vi "Wait.Gui.Open.vi"(6 "Delay at open [ms]":u32, 8 "error in (no error)":errorcluster, 9 "ProgBarSize (0)":i32, 10 "Status (\"\")":string, 11 "Msg":string) -> (0 "error out":errorcluster)   [LabVIEW 2016]
uses:
  Wait.Gui.Action.ctl
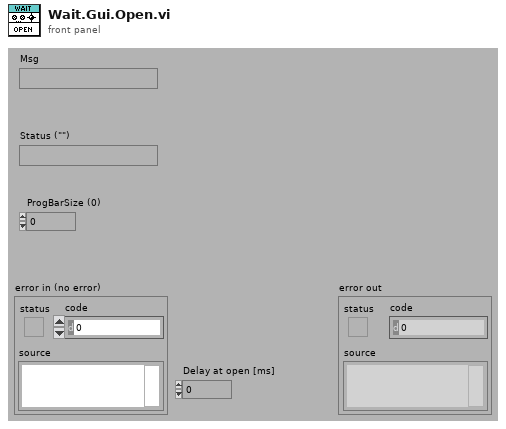
[diagram p1: front panel]
types:
  T1 = typedef "Wait.Gui.Action.ctl" = enum32{"idle", "constructor", "destructor", "--- WaitGui ---", "open FP", "close FP", "update msg", "update progbar"}
  T2 = cluster{"Msg":string, "Status (\"\")":string, "ProgBarSize (0)":i32, "Delay at open [ms]":u32}
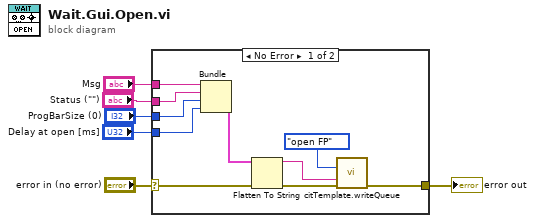
[diagram p0: block diagram]
diagram:
  n1 = case shown="No Error" "error in (no error)" {
    selector: "error in (no error)" -> [w9 w17]
    tunnel: [w16 w17] -> w6
    tunnel: "Msg" -> [w12 _]
    tunnel: "Status (\"\")" -> [w11 _]
    tunnel: "ProgBarSize (0)" -> [w8 _]
    tunnel: "Delay at open [ms]" -> [w7 _]
    frame No Error {
      n2 = Bundle("Msg"=w12, "Status (\"\")"=w11, "ProgBarSize (0)"=w8, "Delay at open [ms]"=w7) -> (w10:T2)  [unwired: 1 in]
      n3 = Flatten To String(anything=w10, error in (no error)=w9) -> (data string=w14:string, error out=w13:errorcluster)  [unwired: 2 in, 1 out]
      n4 = call "citTemplate.writeQueue.vi"("event in (if not connected:all statemachine with data event)"=Wait.Gui.Action."open FP" ("Action"), "data in"=w14, "error in (no error)"=w13) -> ("error out"=w16:errorcluster)  [unwired: 12 in]
    }
    frame Error {
    }
  }
  "error out" <- w6
